vi "GetAllModules.vi"(11 "device in":T1) -> (2 "all modules":string[](array[string]), 3 "device out":T1)   [LabVIEW 2017, in "DeviceModelHelpers.lvlib"]
doc: "Returns the model numbers, such as NI 9205, of every I/O module in the device chassis."
uses:
  <vilib>/addons/InsightCM/Utilities/DeviceModelHelpers/DeviceModelHelpers.lvlib
  <vilib>/addons/InsightCM/MessageBus/Base/controls/R2_Device.ctl
  <vilib>/addons/InsightCM/MessageBus/Base/controls/KeyValuePair.ctl
  <vilib>/addons/InsightCM/MessageBus/Base/controls/DeviceState.ctl
  <vilib>/addons/InsightCM/MessageBus/Base/controls/R2_DataGroup.ctl
  <vilib>/addons/InsightCM/MessageBus/Base/controls/OperatingState.ctl
  <vilib>/addons/InsightCM/MessageBus/Base/controls/Trigger.ctl
  <vilib>/addons/InsightCM/MessageBus/Base/controls/Condition.ctl
  <vilib>/addons/InsightCM/MessageBus/Base/controls/BurstModeTrigger.ctl
  <vilib>/addons/InsightCM/Utilities/PropertyHelpers/PropertyHelpers.lvlib
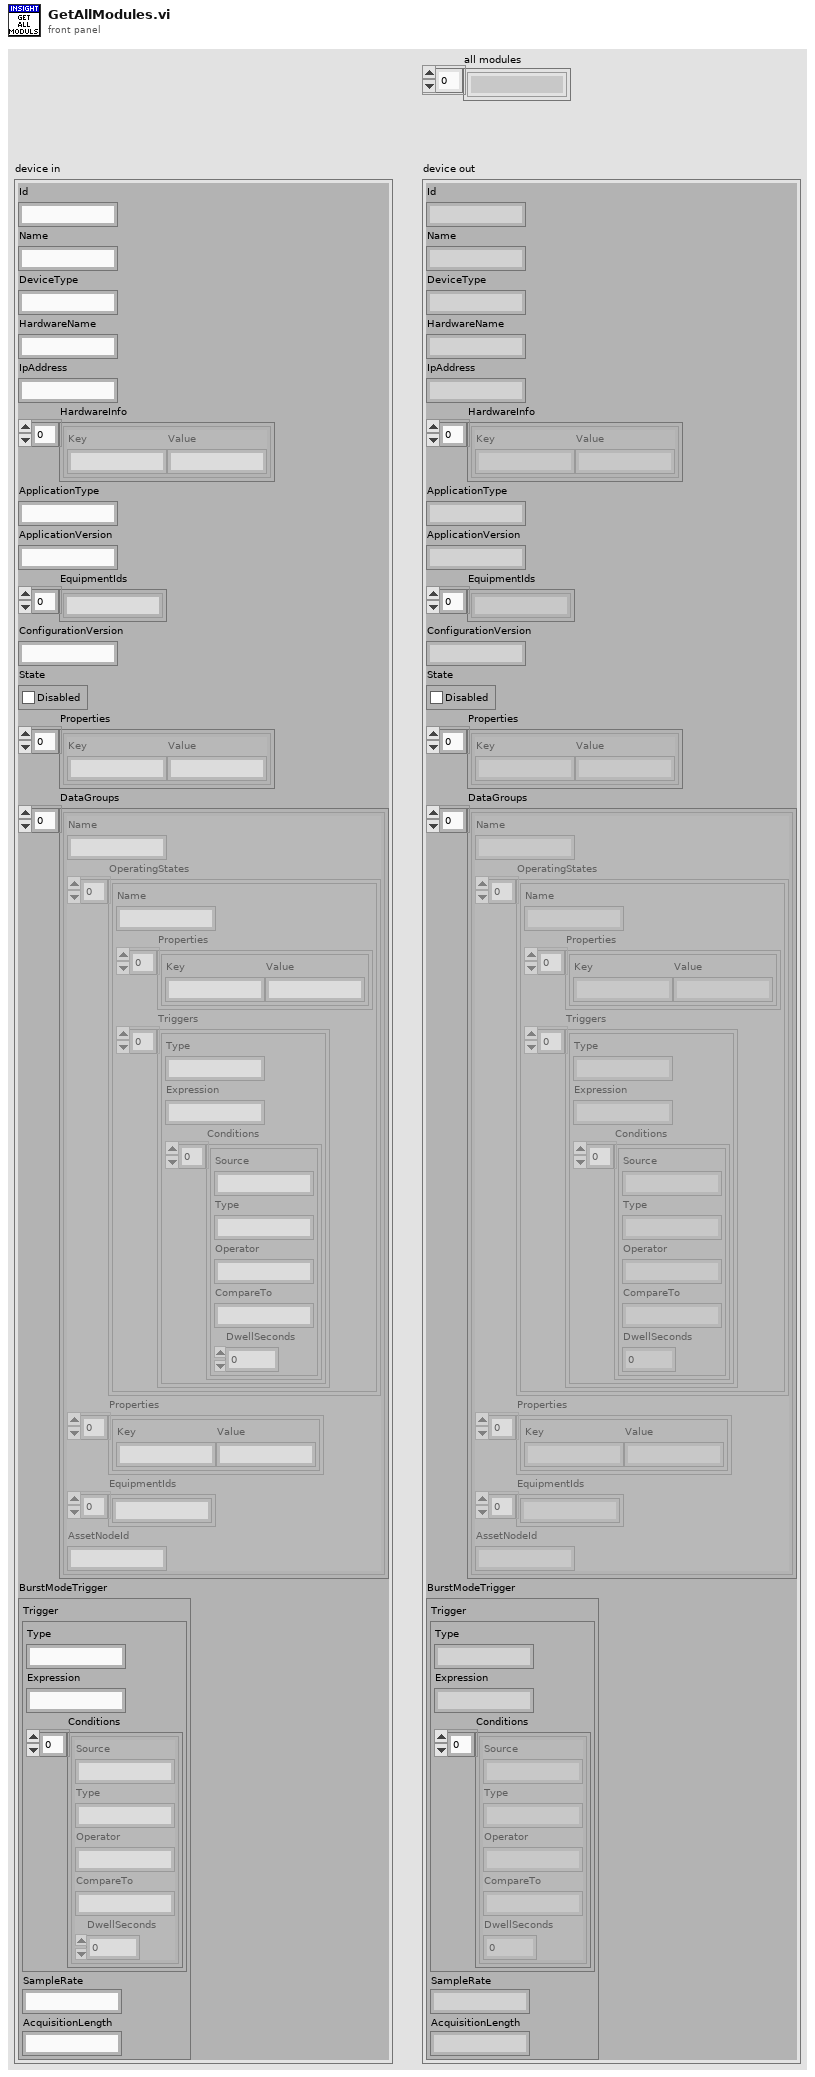
[diagram p1: front panel]
types:
  T1 = typedef "R2_Device.ctl" = cluster{"Id":string, "Name":string, "DeviceType":string, "HardwareName":string, "IpAddress":string, "HardwareInfo":T2[], "ApplicationType":string, "ApplicationVersion":string, "EquipmentIds":string[], "ConfigurationVersion":string, "State":T3, "Properties":T2[], "DataGroups":T4[], "BurstModeTrigger":T8}
  T2 = typedef "KeyValuePair.ctl" = cluster{"Key":string, "Value":string}
  T3 = typedef "DeviceState.ctl" = cluster{"Disabled":bool}
  T4 = typedef "R2_DataGroup.ctl" = cluster{"Name":string, "OperatingStates":T5[], "Properties":T2[], "EquipmentIds":string[], "AssetNodeId":string}
  T5 = typedef "OperatingState.ctl" = cluster{"Name":string, "Properties":T2[], "Triggers":T6[]}
  T6 = typedef "Trigger.ctl" = cluster{"Type":string, "Expression":string, "Conditions":T7[]}
  T7 = typedef "Condition.ctl" = cluster{"Source":string, "Type":string, "Operator":string, "CompareTo":string, "DwellSeconds":dbl}
  T8 = typedef "BurstModeTrigger.ctl" = cluster{"Trigger":T6, "SampleRate":string, "AcquisitionLength":string}
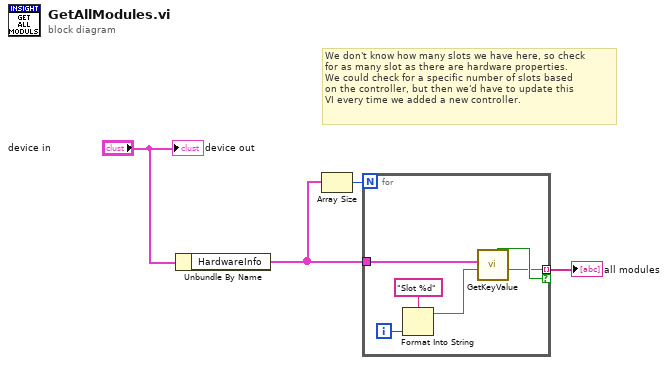
[diagram p0: block diagram]
diagram:
  # "We don't know how many slots we have here, so check\nfor as many slot as there are hardware properties. \nWe could check for a specific number of slots based \non the controller, but then we'd have to update this \nVI every time we added a new controller."
  n1 = Unbundle By Name("device in") -> ("HardwareInfo"=w1:T2[])
  n2 = Array Size(array=w1) -> (size(s)=w4:i32)
  n3 = for {
    N: w4 -> [_]
    tunnel: w1 -> [w7]
    tunnel: [w6] -> w3 mode=indexing if=w8
    i -> [w9]
    n4 = Format Into String(format string="Slot %d", w9) -> (resulting string=w5:string)  [unwired: 2 in, 1 out]
    n5 = call <vilib>:"GetKeyValue.vi"("key"=w5, "key value pairs"=w7) -> ("value"=w6:string, "found"=w8:bool)  [unwired: 7 in, 1 out]
  }
  "all modules" <- w3
  "device out" <- "device in"
